vi "Has All samples.vi"(8 "error in (no error)":errorcluster, 11 "Automation in":refnum<class "NMR Data.lvclass">) -> (0 "error out":errorcluster, 2 "Has all samples?":bool, 3 "Automation out":refnum<class "NMR Data.lvclass">)   [LabVIEW 2019, in "NMR Data.lvclass"]
uses:
  NMR Data.lvclass
  NMR Data.lvclass/NMR Data.ctl
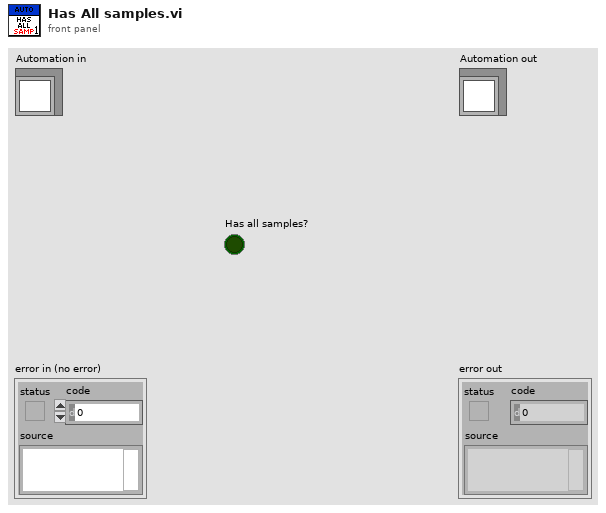
[diagram p1: front panel]
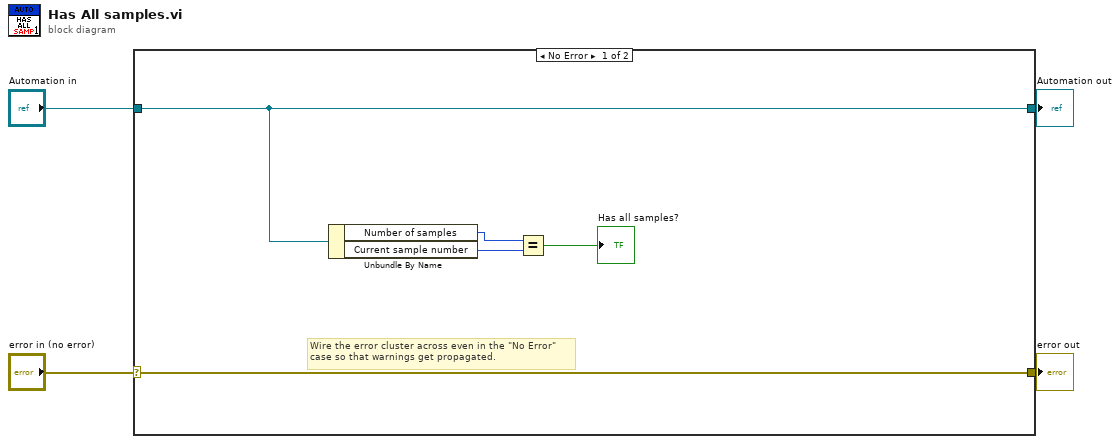
[diagram p0: block diagram]
diagram:
  n1 = case shown="No Error" "error in (no error)" {
    selector: "error in (no error)" -> [w9 w11]
    tunnel: [w9 w11] -> w3
    tunnel: [w5 w10] -> w1
    tunnel: "Automation in" -> [w5 w10]
    frame No Error {
      # "Wire the error cluster across even in the \"No Error\"\ncase so that warnings get propagated."
      n2 = Unbundle By Name(w5) -> ("Number of samples"=w8:i32, "Current sample number"=w7:i32)
      n3 = Equal?(x=w8, y=w7) -> (x = y?=→"Has all samples?":bool)
    }
    frame Error {
    }
  }
  "error out" <- w3
  "Automation out" <- w1
